vi "Input-VMP_TestStand.vi"() -> ()   [LabVIEW 2016]
panel:
  out "Reports Path":path
  out "um/Pixel":dbl format="%#_13g"
  out "Calibration Results File":path
  out "Virtual Stave Map":path
  in  "Calibration Directory":path
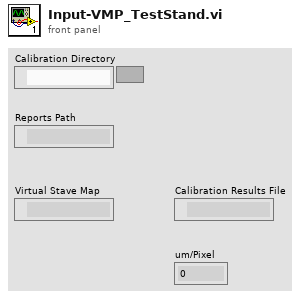
[diagram p1: front panel]
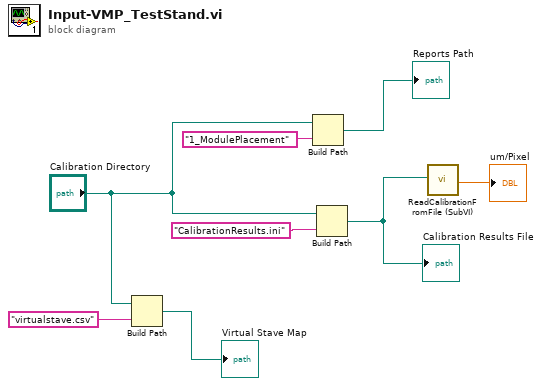
[diagram p0: block diagram]
diagram:
  n1 = Build Path(base path="Calibration Directory", name or relative path="virtualstave.csv") -> (appended path=→"Virtual Stave Map":path)
  n2 = Build Path(base path="Calibration Directory", name or relative path="1_ModulePlacement") -> (appended path=→"Reports Path":path)
  n3 = Build Path(base path="Calibration Directory", name or relative path="CalibrationResults.ini") -> (appended path=w5:path)
  "Calibration Results File" <- w5
  n4 = call "ReadCalibrationFromFile (SubVI).vi"("Calibration file path"=w5) -> ("um/Pixel"=→"um/Pixel":dbl)  [unwired: 12 in, 6 out]
